vi "Flywheel_Execute.vi"() -> ()   [LabVIEW 2019]
uses:
  Globals/Flywheel_Globals.vi
  <vilib>/Rock Robotics/WPI/ThirdParty/REV Robotics/SPARK MAX/Typedef/Spark MAX Control Type.ctl
panel:
  in  "flywheel_max_speed":dbl
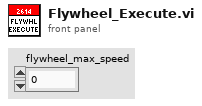
[diagram p1: front panel]
types:
  T1 = typedef "WPI_MotorControlDeviceRef.ctl" = cluster{"DeviceStatus":errorcluster, "Type":T2, "PWM":cluster{"PWM Channel":T3, "DeadBand":T4}, "CAN":cluster{"Device Number":u8, "SetOutput VI Ref":variant, "GetOutput VI Ref":variant, "Enable VI Ref":variant, "Disable VI Ref":variant, "Data":variant}, "Invert":bool, "DIO PWM":cluster{"PWM \"Enable\" Channel":T3, "DIOChannel":T5, "PWM Rate":dbl}}
  T2 = typedef "WPI_MotorControlType.ctl" = enum16{"PWM", "CAN", "DIO PWM"}
  T3 = typedef "FPGA_DIOPWMChannel.ctl" = enum8{"PWM 0", "PWM 1", "PWM 2", "PWM 3", "PWM 4", "PWM 5", "PWM 6", "PWM 7", "PWM 8", "PWM 9", "PWM MXP 0", "PWM MXP 1", "PWM MXP 2", "PWM MXP 3", "PWM MXP 4", "PWM MXP 5", "PWM MXP 6", "PWM MXP 7", "PWM MXP 8", "PWM MXP 9", "Invalid"}
  T4 = typedef "WPI_PWMDeadband.ctl" = cluster{"Name":string, "maxPositivePwm":i32, "minPositivePwm":i32, "centerPwm":i32, "maxNegativePwm":i32, "minNegativePwm":i32, "angularRange":u16}
  T5 = typedef "FPGA_DIOChannel.ctl" = enum8{"DIO 0", "DIO 1", "DIO 2", "DIO 3", "DIO 4", "DIO 5", "DIO 6", "DIO 7", "DIO 8", "DIO 9", "DIO MXP 0", "DIO MXP 1", "DIO MXP 2", "DIO MXP 3", "DIO MXP 4", "DIO MXP 5", "DIO MXP 6", "DIO MXP 7", "DIO MXP 8", "DIO MXP 9", "DIO MXP 10", "DIO MXP 11", "DIO MXP 12", "DIO MXP 13", "DIO MXP 14", "DIO MXP 15", "SPI Port CS1", "SPI Port CS2", "SPI Port CS3", "SPI Port MISO", "SPI Port MOSI", "Invalid"}
  T6 = typedef "Spark MAX Control Type.ctl" = enum16{"Percent VBus", "Voltage", "Velocity", "Position", "Smart Motion", "Current", "Smart Velocity"}
  T7 = typedef "Flywheel_Cluster.ctl" = cluster{"Flywheel_Throttle":dbl, "Control_States":T8, "Auto_Speed":bool, "Flywheel_On":bool}
  T8 = typedef "Flywheel_States.ctl" = enum16{"No-Op", "Percent_Voltage", "Speed_Control_Manual", "Speed_Control_Auto"}
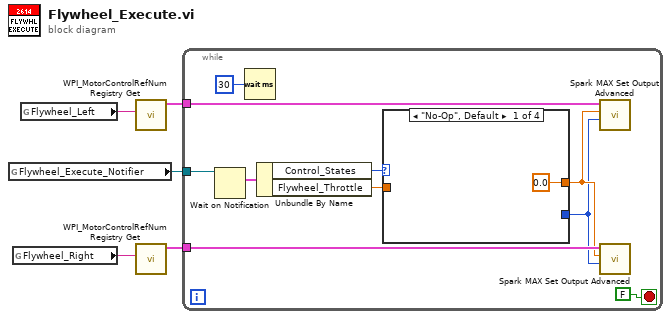
[diagram p0: block diagram]
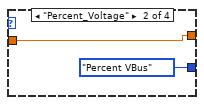
[diagram p2: hidden frame]
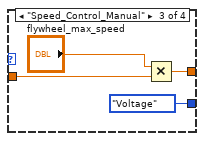
[diagram p3: hidden frame]
diagram:
  n1 = global read "Flywheel_Globals.vi" "Flywheel_Execute_Notifier"() -> (w5:refnum<notifier>)
  n2 = global read "Flywheel_Globals.vi" "Flywheel_Right"() -> (w4:string)
  n3 = global read "Flywheel_Globals.vi" "Flywheel_Left"() -> (w3:string)
  n4 = call <vilib>:"WPI_MotorControlRefNum Registry Get.vi"("refnum name"=w3) -> ("MotorControlDevRef"=w2:T1)  [unwired: 9 in, 1 out]
  n5 = call <vilib>:"WPI_MotorControlRefNum Registry Get.vi"("refnum name"=w4) -> ("MotorControlDevRef"=w1:T1)  [unwired: 9 in, 1 out]
  n6 = while {
    tunnel: w5 -> [w14]
    tunnel: w2 -> [w9]
    tunnel: w1 -> [w8]
    stop <- FALSE stop-if-true
    n7 = Wait on Notification(notifier=w14) -> (notification=w13:T7)  [unwired: 3 in, 3 out]
    n8 = Wait (ms)(milliseconds to wait=u32 30) -> ()  [unwired: 1 out]
    n9 = Unbundle By Name(w13) -> ("Control_States"=w12:T8, "Flywheel_Throttle"=w11:dbl)
    n10 = case shown="\"No-Op\", Default" w12 {
      tunnel: [0.0 ("Flywheel_Throttle") w18 w22 _] -> w7
      tunnel: w11 -> [_ w18 w21 _]
      tunnel: [_ Spark_MAX_Control_Type."Percent VBus" ("Control Mode") Spark_MAX_Control_Type."Voltage" ("Control Mode") _] -> w6
      frame "No-Op", Default {
      }
      frame "Percent_Voltage" {
      }
      frame "Speed_Control_Manual" {
        n11 = Multiply(x="flywheel_max_speed", y=w21) -> (x*y=w22:dbl)
      }
      frame "Speed_Control_Auto" {
        # "fancy speed control logic"
      }
    }
    n12 = call <vilib>:"Spark MAX Set Output Advanced.vi"("Control Mode"=w6, "Setpoint"=w7, "MotorControlDevRef"=w9) -> ()  [unwired: 7 in, 2 out]
    n13 = call <vilib>:"Spark MAX Set Output Advanced.vi"("Control Mode"=w6, "Setpoint"=w7, "MotorControlDevRef"=w8) -> ()  [unwired: 7 in, 2 out]
  }
